vi "基础9.vi"() -> ()   [LabVIEW 2014]
panel:
  out "布尔 5":bool
  out "布尔 4":bool
  out "布尔 3":bool
  out "布尔 2":bool
  out "布尔":bool
  in  "停止":bool
  in  "滑动杆":dbl(slide) scale=0.0..500.0
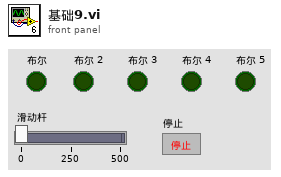
[diagram p1: front panel]
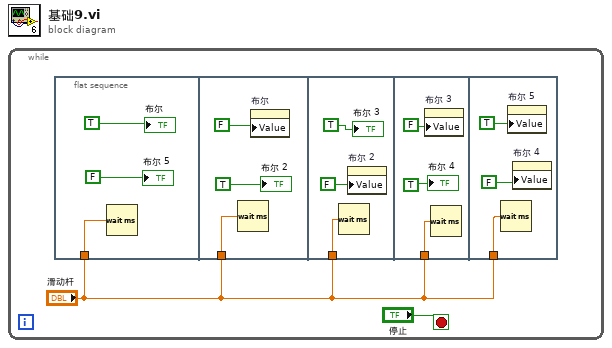
[diagram p0: block diagram]
diagram:
  n1 = while {
    stop <- "停止" stop-if-true
    n2 = flat-sequence {
      tunnel: "滑动杆" -> [w5]
      tunnel: "滑动杆" -> [w8]
      tunnel: "滑动杆" -> [w11]
      tunnel: "滑动杆" -> [w14]
      tunnel: "滑动杆" -> [w17]
      frame #0 {
        n3 = Wait (ms)(milliseconds to wait=w5) -> ()  [unwired: 1 out]
        "布尔 5" <- FALSE
        "布尔" <- TRUE
      }
      frame #1 {
        n4 = Wait (ms)(milliseconds to wait=w8) -> ()  [unwired: 1 out]
        n5 = property on="布尔" class="Bool (严格)"("Value"=FALSE) -> ()  [unwired: 2 in, 2 out]
        "布尔 2" <- TRUE
      }
      frame #2 {
        n6 = Wait (ms)(milliseconds to wait=w11) -> ()  [unwired: 1 out]
        n7 = property on="布尔 2" class="Bool (严格)"("Value"=FALSE) -> ()  [unwired: 2 in, 2 out]
        "布尔 3" <- TRUE
      }
      frame #3 {
        n8 = property on="布尔 3" class="Bool (严格)"("Value"=FALSE) -> ()  [unwired: 2 in, 2 out]
        n9 = Wait (ms)(milliseconds to wait=w14) -> ()  [unwired: 1 out]
        "布尔 4" <- TRUE
      }
      frame #4 {
        n10 = Wait (ms)(milliseconds to wait=w17) -> ()  [unwired: 1 out]
        n11 = property on="布尔 5" class="Bool (严格)"("Value"=TRUE) -> ()  [unwired: 2 in, 2 out]
        n12 = property on="布尔 4" class="Bool (严格)"("Value"=FALSE) -> ()  [unwired: 2 in, 2 out]
      }
    }
  }
